vi "Init Active Device Array.vi"(8 "error in":errorcluster, 11 "DAC TC Temperature in":refnum<class "DAC TC Temperature.lvclass">) -> (0 "error out":errorcluster, 2 "Active Device Array":bool[](array[boolean]), 3 "DAC TC Temperature out":refnum<class "DAC TC Temperature.lvclass">)   [LabVIEW 2019, in "DAC.lvlib" / "DAC TC Temperature.lvclass"]
uses:
  DAC TC Temperature.lvclass
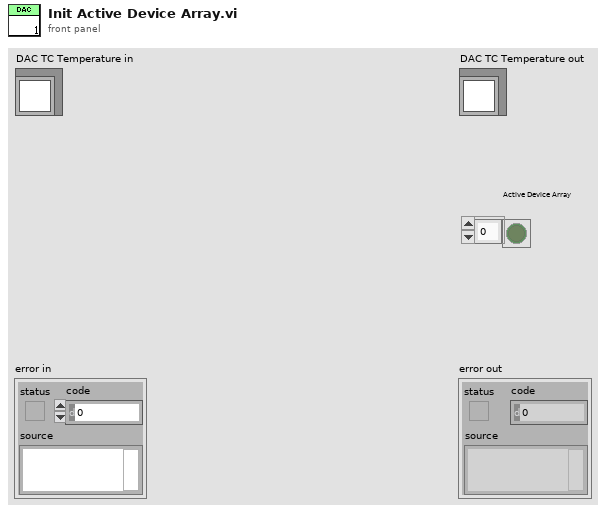
[diagram p1: front panel]
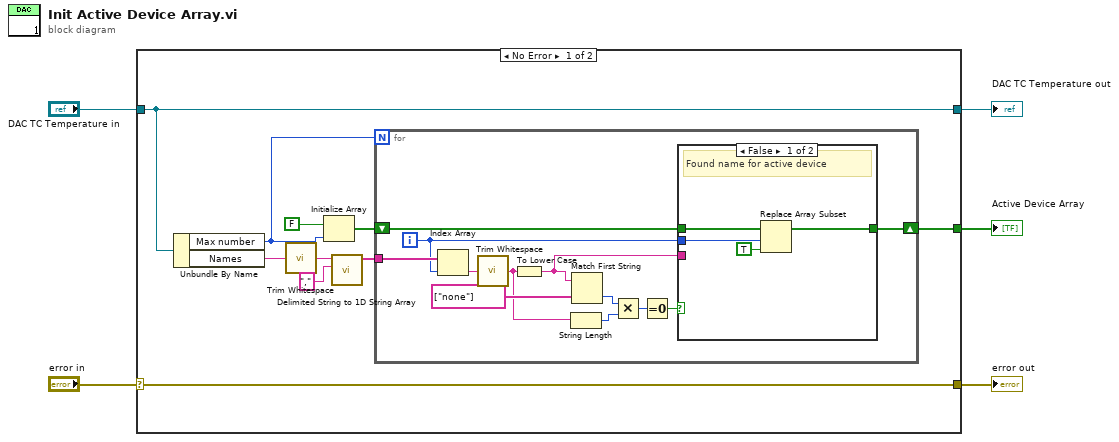
[diagram p0: block diagram]
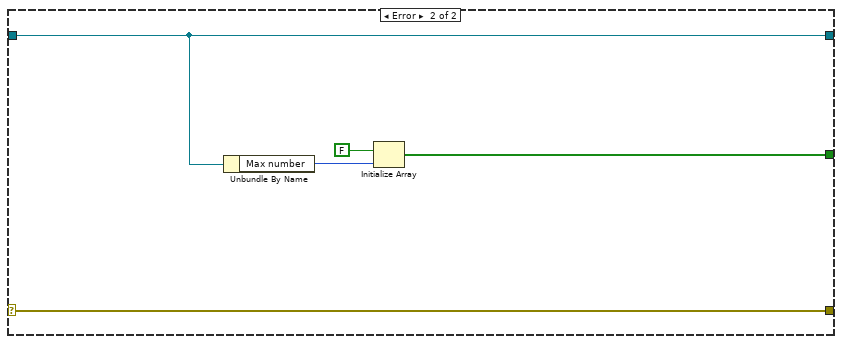
[diagram p3: hidden frame]
diagram:
  n1 = case shown="No Error" "error in" {
    selector: "error in" -> [w6 w37]
    tunnel: [w6 w37] -> w4
    tunnel: [w15 w34] -> w2
    tunnel: "DAC TC Temperature in" -> [w15 w34]
    tunnel: [w7 w33] -> w1
    frame No Error {
      n2 = Unbundle By Name(w15) -> ("Max number"=w9:i32, "Names"=w14:string)
      n3 = call <vilib>:"Trim Whitespace.vi"("string"=w14) -> ("trimmed string"=w13:string)  [unwired: 1 in]
      n4 = Initialize Array(FALSE, w9) -> (w8:bool[])
      n5 = call <vilib>:"Delimited String to 1D String Array.vi"("delimiter"=",", "delimited string"=w13) -> ("string array"=w10:string[])  [unwired: 9 in]
      n6 = for {
        N: w9 -> [_]
        tunnel: w10 -> [w27]
        shift-right: [w16] -> w7
        shift-left: w8 -> [w17]
        i -> [w18]
        n7 = Index Array(array=w27, index=w18) -> (element=w26:string)
        n8 = call <vilib>:"Trim Whitespace.vi"("string"=w26) -> ("trimmed string"=w23:string)  [unwired: 1 in]
        n9 = To Lower Case(string=w23) -> (all lower case string=w25:string)
        n10 = String Length(string=w23) -> (length=w22:i32)
        n11 = Match First String(2:string[] ["none"], 3:w25) -> (0:w21:i32)  [unwired: 1 out]
        n12 = Multiply(x=w21, y=w22) -> (x*y=w20:i32)
        n13 = Equal To 0?(x=w20) -> (x = 0?=w19:bool)
        n14 = case shown="False" w19 {
          tunnel: w25 -> [_ _]
          tunnel: w18 -> [w30 _]
          tunnel: w17 -> [w31 w32]
          tunnel: [w28 w32] -> w16
          frame False {
            # "Found name for active device"
            n15 = Replace Array Subset "Replace Array Subset"(array=w31, new element=TRUE ("new element/subarray"), index=w30) -> (w28:bool[])
          }
          frame True {
            # "Empty or 'none' - inactive device"
          }
        }
      }
    }
    frame Error {
      n16 = Unbundle By Name(w34) -> ("Max number"=w35:i32)
      n17 = Initialize Array(FALSE, w35) -> (w33:bool[])
    }
  }
  "error out" <- w4
  "DAC TC Temperature out" <- w2
  "Active Device Array" <- w1
